vi "DAQSpeedCalc (1).vi"(11 "Distance":dbl) -> (3 "Speed":dbl)   [LabVIEW 2017]
uses:
  <vilib>/Analysis/baseanly.llb/Mean (DBL).vi
  LoopPeriodGLOBAL.vi
  <vilib>/Analysis/NI_AALBase.lvlib
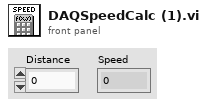
[diagram p1: front panel]
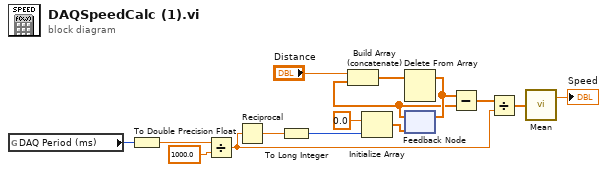
[diagram p0: block diagram]
diagram:
  n1 = global read "LoopPeriodGLOBAL.vi" "DAQ Period (ms)"() -> (w13:u32)
  n2 = To Double Precision Float(number=w13) -> (double precision float=w11:dbl)
  n3 = Divide(x=w11, y=1000.0) -> (x/y=w5:dbl)
  n4 = Reciprocal(x=w5) -> (1/x=w4:dbl)
  n5 = To Long Integer(number=w4) -> (32bit integer=w2:i32)
  n6 = Initialize Array(0.0 ("element"), w2) -> (w1:dbl[])
  n7 = feedback #1(w1) -> (w7:dbl[])
  n8 = Build Array (concatenate)("Distance", w7) -> (w15:dbl[])
  n9 = Delete From Array(array=w15) -> (array with subset deleted=w8:dbl[])  [unwired: 2 in, 1 out]
  n10 = feedback-in #1(w8) -> ()
  n11 = Subtract(x=w8, y=w7) -> (x-y=w14:dbl[])
  n12 = Divide(x=w14, y=w5) -> (x/y=w10:dbl[])
  n13 = call-poly <vilib>:"Mean.vi"("X"=w10) -> ("mean"=→"Speed":dbl)  [unwired: 1 out]
